vi "Background.vi"() -> (0 "?":picture)   [LabVIEW 2014]
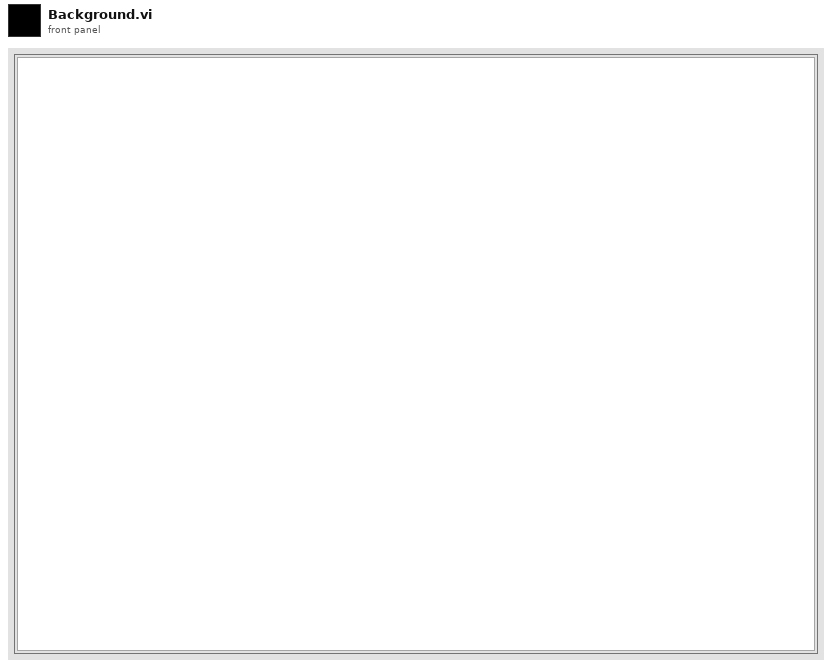
[diagram p1: front panel]
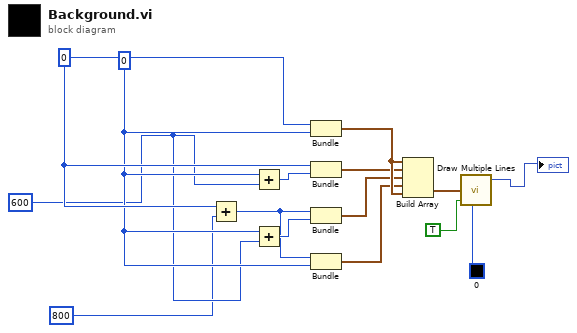
[diagram p0: block diagram]
diagram:
  w7 = i16 0 ("Origin Y")
  w12 = i16 0 ("Origin X")
  w2 = i16 600 ("Height")
  n1 = Add(x=w12, y=i16 800 ("Width")) -> (x+y=w8:i16)
  n2 = Add(x=w7, y=w2) -> (x+y=w11:i16)
  n3 = Add(x=w7, y=w2) -> (x+y=w9:i16)
  n4 = Bundle("Origin X"=w12, "Origin Y"=w7) -> (w15:cluster{"Origin X":i16, "Origin Y":i16})  [unwired: 1 in]
  n5 = Bundle("Origin X"=w12, w11) -> (w13:cluster{"Origin X":i16, i16})  [unwired: 1 in]
  n6 = Bundle(w8, w9) -> (w10:cluster{i16, i16})  [unwired: 1 in]
  n7 = Bundle(w8, "Origin Y"=w7) -> (w6:cluster{i16, "Origin Y":i16})  [unwired: 1 in]
  n8 = Build Array(w15, w13, w10, w6, w15) -> (w14:cluster{"Origin X":i16, "Origin Y":i16}[])
  n9 = call <vilib>:"Draw Multiple Lines.vi"("line endpoints"=w14, "fill?(F)"=TRUE, "color(black)"=u32 0) -> ("new picture"=→"?":picture)  [unwired: 6 in]
